vi "LWXPS_GetCurrentPosition.vi"(0 "XPS Reference IN":refnum<k24>, 5 "LabVIEW error IN":errorcluster) -> (10 "XPS Reference OUT":refnum<k24>, 11 "LabVIEW error OUT":errorcluster, 12 "Returned error code":i32, 13 "XPS Error String":string, 14 "Y Position in µm":dbl, 15 "X Position in µm":dbl, 16 "X1 Position counts":i32, 17 "X2 Position counts":i32, 18 "Y Laser Position counts":i32, 19 "X Laser Position counts":i32)   [LabVIEW 2014]
uses:
  D:/XPSQ8_LabView_Library/Development/Source/Dll/Newport.XPS.CommandInterface.dll
  Dll/Newport.XPS.CommandInterface.dll
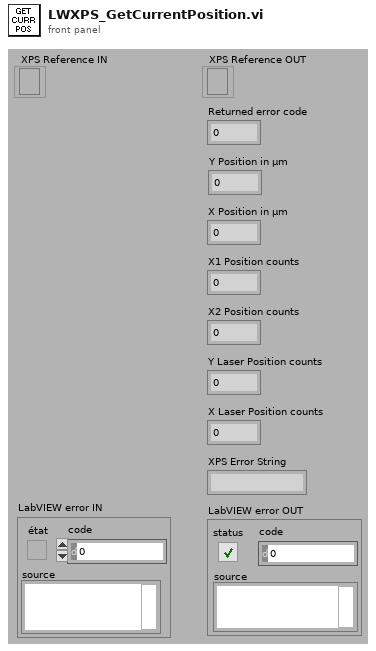
[diagram p1: front panel]
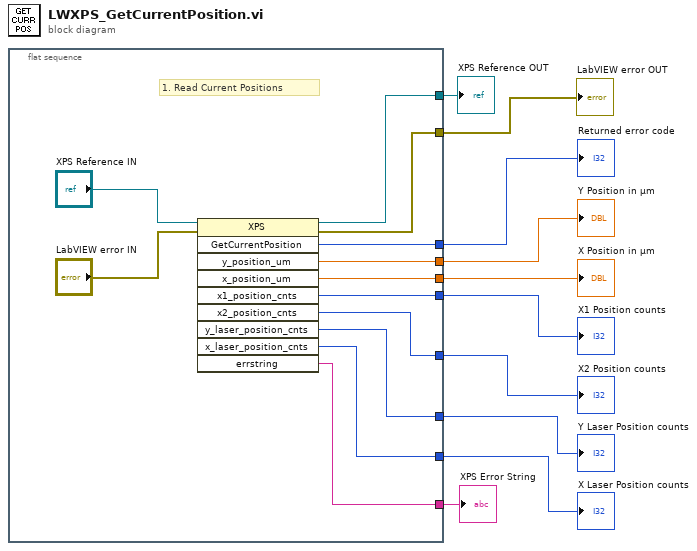
[diagram p0: block diagram]
diagram:
  n1 = flat-sequence {
    tunnel: [w21] -> w10
    tunnel: [w20] -> w6
    tunnel: [w19] -> w9
    tunnel: [w15] -> w4
    tunnel: [w18] -> w5
    tunnel: [w17] -> w8
    tunnel: [w16] -> w7
    tunnel: [w13] -> w1
    tunnel: [w14] -> w2
    tunnel: [w12] -> w3
    frame #0 {
      # "1. Read Current Positions"
      n2 = invoke class="XPS" method="GetCurrentPosition"(reference="XPS Reference IN", error in="LabVIEW error IN") -> (reference out=w21:refnum<k24>, error out=w20:errorcluster, "GetCurrentPosition"=w12:i32, "y_position_um"=w15:dbl, "x_position_um"=w18:dbl, "x1_position_cnts"=w17:i32, "x2_position_cnts"=w16:i32, "y_laser_position_cnts"=w13:i32, "x_laser_position_cnts"=w14:i32, "errstring"=w19:string)  [unwired: 8 in]
    }
  }
  "XPS Reference OUT" <- w10
  "LabVIEW error OUT" <- w6
  "XPS Error String" <- w9
  "Y Position in µm" <- w4
  "X Position in µm" <- w5
  "X1 Position counts" <- w8
  "X2 Position counts" <- w7
  "Y Laser Position counts" <- w1
  "X Laser Position counts" <- w2
  "Returned error code" <- w3
